vi "pi_to_180.vi"(10 "起始角度":dbl, 11 "输入角度":sgl) -> (3 "数值":dbl)   [LabVIEW 2016]
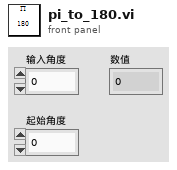
[diagram p1: front panel]
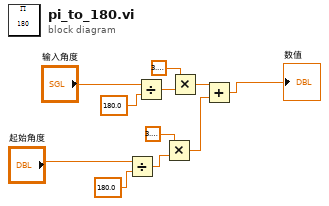
[diagram p0: block diagram]
diagram:
  n1 = Divide(x="起始角度", y=180.0) -> (x/y=w5:dbl)
  n2 = Divide(x="输入角度", y=180.0) -> (x/y=w2:dbl)
  n3 = Multiply(x=3.141592653589793, y=w5) -> (x*y=w7:dbl)
  n4 = Multiply(x=3.141592653589793, y=w2) -> (x*y=w3:dbl)
  n5 = Add(x=w3, y=w7) -> (x+y=→"数值":dbl)
